vi "Word_Set_Selection_Borders.vi"(0 "Word.Selection":refnum<k7>, 7 "borders and shading":T1={"outside line style"=1, "outside color"=4278190080, "outside line width"=2, "inside line style"=1, "inside color"=4278190080, "inside line width"=2, "background pattern color"=4278190080} {"inside line style" items=["wdLineStyleNone", "wdLineStyleSingle", "wdLineStyleDot", "wdLineStyleDashSmallGap", "wdLineStyleDashLargeGap", "wdLineStyleDashDot", "wdLineStyleDashDotDot", "wdLineStyleDouble", "wdLineStyleTriple", "wdLineStyleThinThickSmallGap", "wdLineStyleThickThinSmallGap", "wdLineStyleThinThickThinSmallGap", "wdLineStyleThinThickMedGap", "wdLineStyleThickThinMedGap", "wdLineStyleThinThickThinMedGap", "wdLineStyleThinThickLargeGap", "wdLineStyleThickThinLargeGap", "wdLineStyleThinThickThinLargeGap", "wdLineStyleSingleWavy", "wdLineStyleDoubleWavy", "wdLineStyleDashDotStroked", "wdLineStyleEmboss3D", "wdLineStyleEngrave3D", "wdLineStyleOutset", "wdLineStyleInset"]; "inside line width" items=["wdLineWidth025pt"=2, "wdLineWidth050pt"=4, "wdLineWidth075pt"=6, "wdLineWidth100pt"=8, "wdLineWidth150pt"=12, "wdLineWidth225pt"=18, "wdLineWidth300pt"=24, "wdLineWidth450pt"=36, "wdLineWidth600pt"=48]; "outside line width" items=["wdLineWidth025pt"=2, "wdLineWidth050pt"=4, "wdLineWidth075pt"=6, "wdLineWidth100pt"=8, "wdLineWidth150pt"=12, "wdLineWidth225pt"=18, "wdLineWidth300pt"=24, "wdLineWidth450pt"=36, "wdLineWidth600pt"=48]; "outside line style" items=["wdLineStyleNone", "wdLineStyleSingle", "wdLineStyleDot", "wdLineStyleDashSmallGap", "wdLineStyleDashLargeGap", "wdLineStyleDashDot", "wdLineStyleDashDotDot", "wdLineStyleDouble", "wdLineStyleTriple", "wdLineStyleThinThickSmallGap", "wdLineStyleThickThinSmallGap", "wdLineStyleThinThickThinSmallGap", "wdLineStyleThinThickMedGap", "wdLineStyleThickThinMedGap", "wdLineStyleThinThickThinMedGap", "wdLineStyleThinThickLargeGap", "wdLineStyleThickThinLargeGap", "wdLineStyleThinThickThinLargeGap", "wdLineStyleSingleWavy", "wdLineStyleDoubleWavy", "wdLineStyleDashDotStroked", "wdLineStyleEmboss3D", "wdLineStyleEngrave3D", "wdLineStyleOutset", "wdLineStyleInset"]}, 11 "error in":errorcluster) -> (15 "error out":errorcluster)   [LabVIEW 2010, in "NI_ReportGenerationToolkit.lvlib"]
uses:
  <vilib>/addons/_office/NI_ReportGenerationToolkit.lvlib
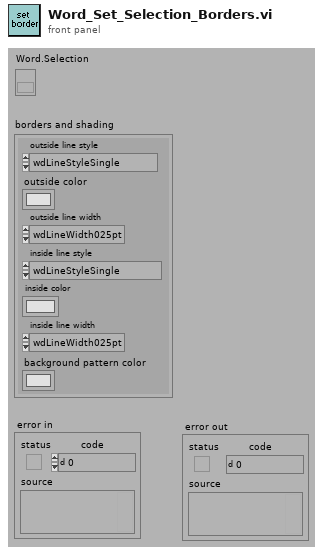
[diagram p1: front panel]
types:
  T1 = cluster{"outside line style":i32, "outside color":u32, "outside line width":i32, "inside line style":i32, "inside color":u32, "inside line width":i32, "background pattern color":u32}
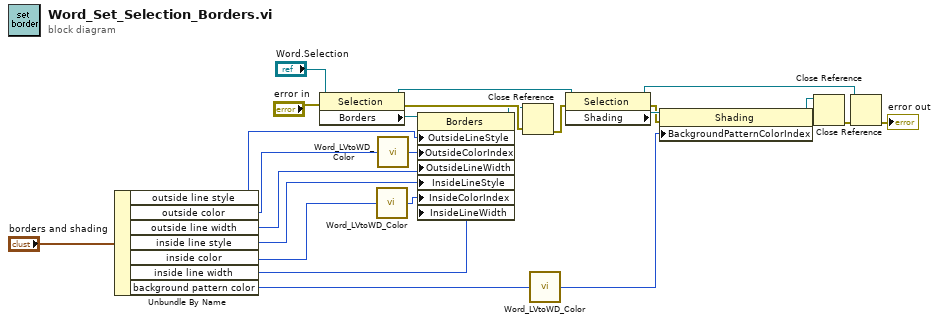
[diagram p0: block diagram]
diagram:
  n1 = Unbundle By Name("borders and shading") -> ("outside line style"=w18:i32, "outside color"=w5:u32, "outside line width"=w17:i32, "inside line style"=w16:i32, "inside color"=w3:u32, "inside line width"=w15:i32, "background pattern color"=w7:u32)
  n2 = property class="Selection"(reference="Word.Selection", error in="error in") -> (reference out=w20:refnum<k7>, error out=w25:errorcluster, "Borders"=w22:refnum<k7>)
  n3 = call <vilib>:"Word_LVtoWD_Color.vi"("LabVIEW color"=w3) -> ("word color table index"=w2:i32)
  n4 = call <vilib>:"Word_LVtoWD_Color.vi"("LabVIEW color"=w5) -> ("word color table index"=w4:i32)
  n5 = property class="Borders"(reference=w22, "OutsideLineStyle"=w18, "OutsideColorIndex"=w4, "OutsideLineWidth"=w17, "InsideLineStyle"=w16, "InsideColorIndex"=w2, "InsideLineWidth"=w15) -> (reference out=w23:refnum<k7>)  [unwired: 1 in, 1 out]
  n6 = Close Reference(reference=w23, error in (no error)=w25) -> (error out=w24:errorcluster)
  n7 = call <vilib>:"Word_LVtoWD_Color.vi"("LabVIEW color"=w7) -> ("word color table index"=w6:i32)
  n8 = property class="Selection"(reference=w20, error in=w24) -> (reference out=w10:refnum<k7>, error out=w8:errorcluster, "Shading"=w19:refnum<k7>)
  n9 = property class="Shading"(reference=w19, error in=w8, "BackgroundPatternColorIndex"=w6) -> (reference out=w12:refnum<k7>, error out=w13:errorcluster)
  n10 = Close Reference(reference=w12, error in (no error)=w13) -> (error out=w11:errorcluster)
  n11 = Close Reference(reference=w10, error in (no error)=w11) -> (error out=→"error out":errorcluster)
